vi "WebSocket FGV.vi"(0 "Tx to Server":string, 5 "Action":T2, 7 "TCP Address":string, 9 "TCP Port":u32, 11 "error in (no error)":errorcluster) -> (3 "Server Info":string, 4 "Rx from Server":string, 8 "Connection Status":bool, 13 "TxStats":T1, 14 "RxStats":T1, 15 "error out":errorcluster)   [LabVIEW 2023]
uses:
  Windows/WebSocket VIG States.ctl
  WebSocket/Stats.ctl
  WebSocket/WebSocket Stats VIG Mode.ctl
  <vilib>/Utility/error.llb/Trim Whitespace One-Sided.vi
  WebSocket/WebSocket.lvclass
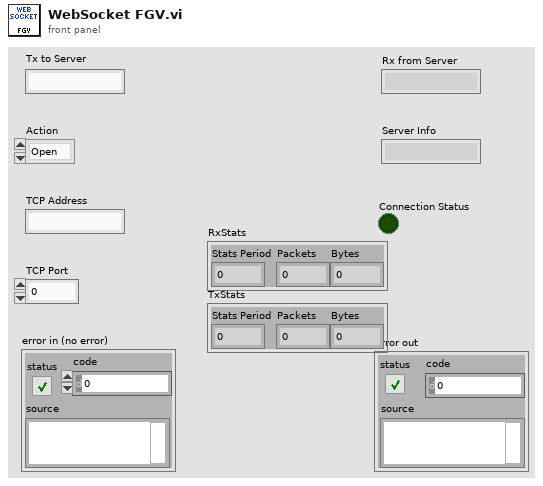
[diagram p1: front panel]
types:
  T1 = typedef "WebSocket.lvclass/Stats.ctl" = cluster{"Stats Period":dbl, "Packets":u64, "Bytes":u64}
  T2 = typedef "WebSocket VIG States.ctl" = enum16{"Open", "Close", "Send", "Receive", "Check"}
  T3 = typedef "WebSocket Stats VIG Mode.ctl" = enum16{"Init", "Set", "Update", "Get All"}
  T4 = enum16{"Standard", "Buffered", "CRLF", "Immediate"}
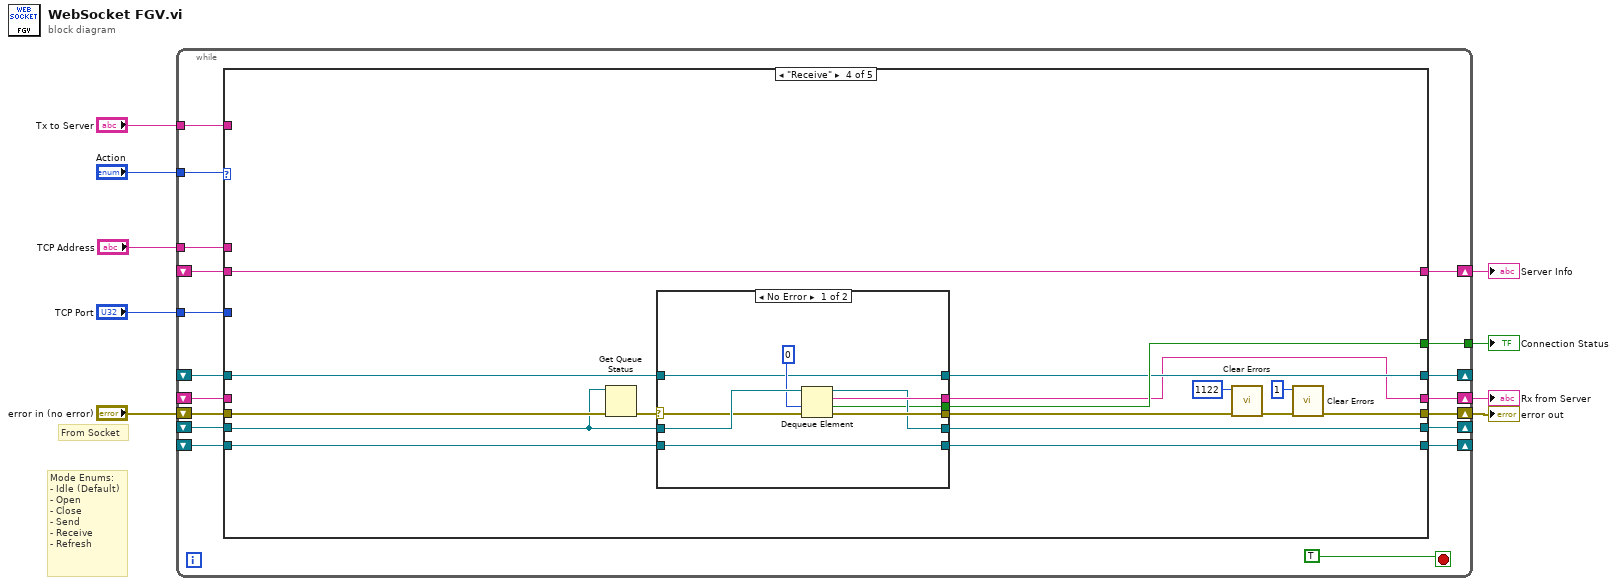
[diagram p0: block diagram]
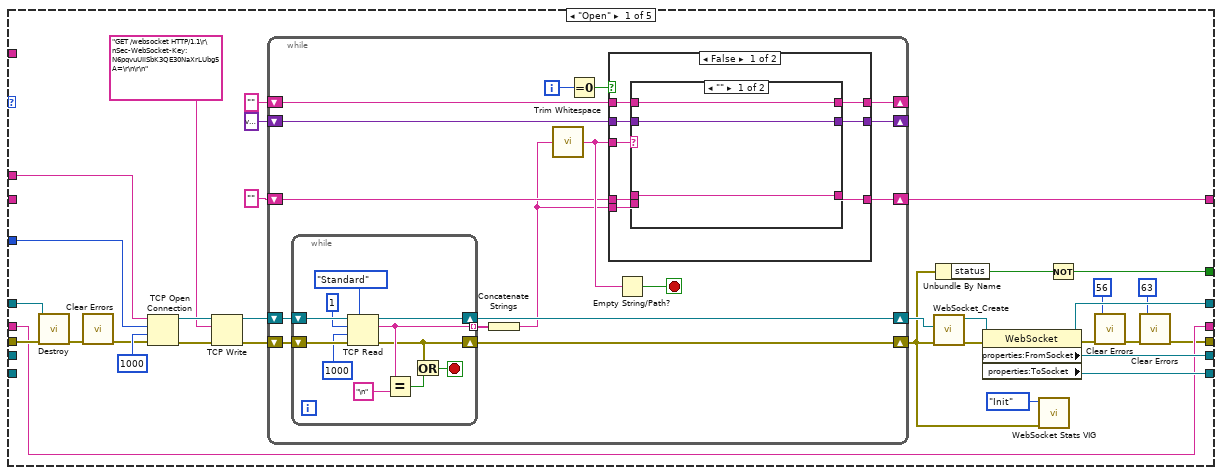
[diagram p2: hidden frame]
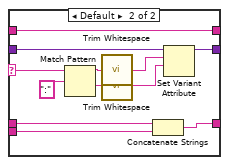
[diagram p3: hidden frame]
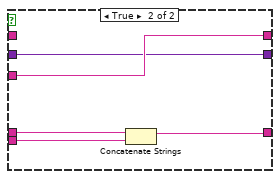
[diagram p4: hidden frame]
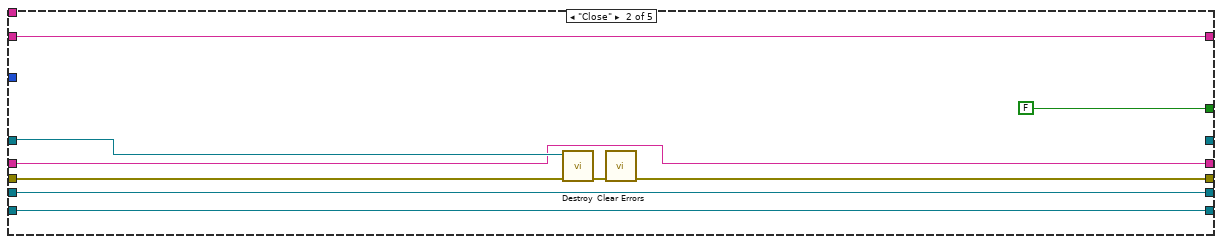
[diagram p5: hidden frame]
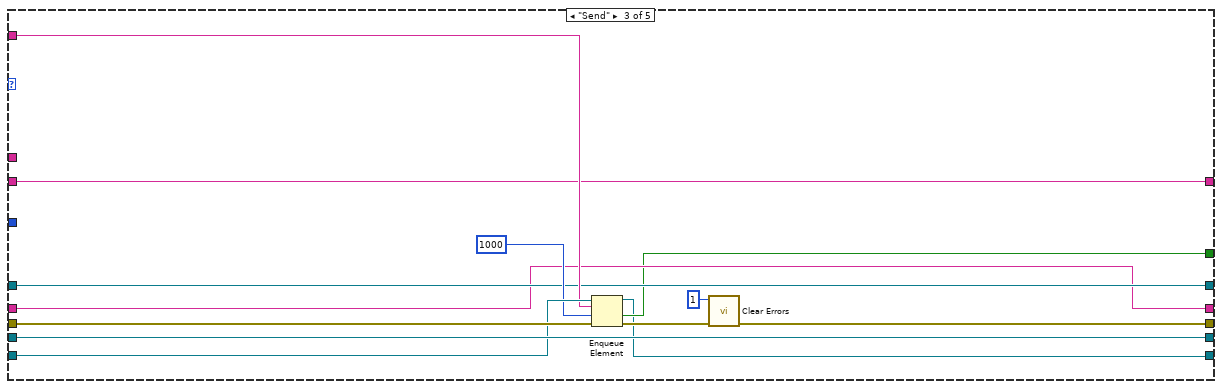
[diagram p6: hidden frame]
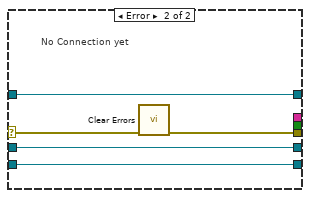
[diagram p7: hidden frame]
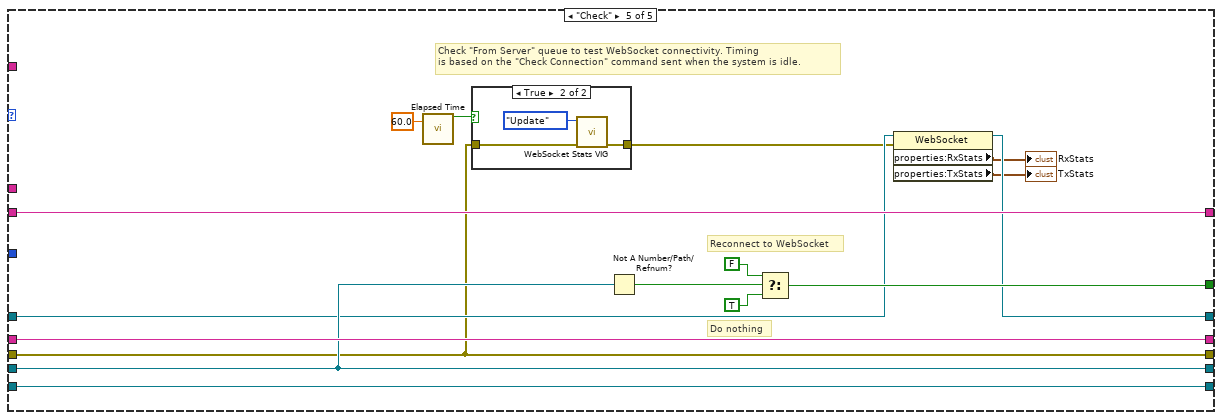
[diagram p8: hidden frame]
diagram:
  # "From Socket"
  # "Mode Enums:\n- Idle (Default)\n- Open\n- Close\n- Send\n- Receive\n- Refresh"
  n1 = while {
    tunnel: "Action" -> [w27]
    tunnel: "TCP Port" -> [w26]
    shift-right: [w24] -> w7
    shift-left: "error in (no error)" -> [w25]
    shift-right: [w23] -> _
    shift-left: _ -> [w16]
    tunnel: "TCP Address" -> [w22]
    shift-right: [w20] -> _
    shift-left: _ -> [w17]
    shift-right: [w19] -> _
    shift-left: _ -> [w18]
    tunnel: "Tx to Server" -> [w14]
    shift-right: [w21] -> w5
    shift-left: _ -> [w13]
    shift-right: [w15] -> w4
    shift-left: _ -> [w12]
    tunnel: [w10] -> w1
    stop <- TRUE stop-if-true
    n2 = case shown="\"Receive\"" w27 {
      tunnel: w26 -> [w49 _ _ _ _]
      tunnel: w25 -> [w48 w123 w135 w148 w168]
      tunnel: [w32 w115 w125 w139 w168] -> w24
      tunnel: [w34 _ w129 w144 w174] -> w23
      tunnel: w22 -> [w46 _ _ _ _]
      tunnel: [w45 w118 w130 w151 w182] -> w21
      tunnel: [w44 w119 w136 w150 w179] -> w20
      tunnel: [w43 w120 w126 w142 w180] -> w19
      tunnel: w18 -> [_ w120 w133 w143 w180]
      tunnel: w17 -> [_ w119 w136 w147 w179]
      tunnel: w16 -> [w37 w121 w129 w145 w173]
      tunnel: [w35 w117 w128 w141 w181] -> w15
      tunnel: w14 -> [_ _ w132 _ _]
      tunnel: w13 -> [_ w118 w130 w151 w182]
      tunnel: w12 -> [w35 w117 w128 _ w181]
      tunnel: [w40 FALSE ("timed out?") w127 w149 w176] -> w10
      frame "Open" {
        n3 = call-dynamic "Destroy.vi"("error in (no error)"=w48, "reference in"=w37) -> ("error out"=w38:errorcluster)  [unwired: 8 in, 1 out]
        n4 = call <vilib>:"Clear Errors.vi"("error in (no error)"=w38) -> ("error out"=w36:errorcluster)  [unwired: 5 in, 1 out]
        n5 = TCP Open Connection(address=w46, remote port or service name=w49, timeout ms (60000)=1000, error in (no error)=w36) -> (connection ID=w51:refnum<k5>, error out=w50:errorcluster)  [unwired: 1 in]
        n6 = TCP Write(connection ID=w51, data in="GET /websocket HTTP/1.1\r\nSec-WebSocket-Key: N6pqvuUIiSbK3QE30NaXrLUbg5A=\r\n\r\n", error in (no error)=w50) -> (connection ID out=w55:refnum<k5>, error out=w56:errorcluster)  [unwired: 1 in, 1 out]
        n7 = while {
          shift-right: [w67] -> _
          shift-left: variant -> [w68]
          shift-right: [w71] -> _
          shift-left: "" ("trimmed string") -> [w70]
          shift-right: [w66] -> w57
          shift-left: w55 -> [w75]
          shift-right: [w65] -> w28
          shift-left: w56 -> [w74]
          shift-right: [w63] -> w45
          shift-left: "" ("trimmed string") -> [w62]
          i -> [w73]
          stop <- w60 stop-if-true
          n8 = while {
            tunnel: [w81] -> w64 mode=indexing
            shift-right: [w82] -> w66
            shift-left: w75 -> [w86]
            shift-right: [w78] -> w65
            shift-left: w74 -> [w85]
            stop <- w77 stop-if-true
            n9 = TCP Read(connection ID=w86, bytes to read=1, error in (no error)=w85, 7:T4."Standard" ("mode (standard)"), 9:1000 ("timeout ms (25000)")) -> (connection ID out=w82:refnum<k5>, data out=w81:string, error out=w78:errorcluster)
            n10 = Equal?(x=w81, y="\n") -> (x = y?=w79:bool)
            n11 = Or(x=w78, y=w79) -> (x .or. y?=w77:bool)
          }
          n12 = Concatenate Strings(w64) -> (w61:string)
          n13 = call <vilib>:"Trim Whitespace.vi"("string"=w61) -> ("trimmed string"=w69:string)  [unwired: 1 in]
          n14 = Equal To 0?(x=w73) -> (x = 0?=w72:bool)
          n15 = case shown="False" w72 {
            tunnel: [w90 w114] -> w71
            tunnel: w69 -> [w92 w114]
            tunnel: w70 -> [w91 _]
            tunnel: w68 -> [w94 w113]
            tunnel: [w93 w113] -> w67
            tunnel: w61 -> [w89 w110]
            tunnel: [w88 w111] -> w63
            tunnel: w62 -> [w87 w112]
            frame False {
              n16 = case shown="\"\"" w92 {
                selector: w92 -> [_ w102]
                tunnel: w94 -> [w97 w106]
                tunnel: [w97 w105] -> w93
                tunnel: w91 -> [w96 w101]
                tunnel: [w96 w101] -> w90
                tunnel: w89 -> [_ w100]
                tunnel: [w95 w99] -> w88
                tunnel: w87 -> [w95 w98]
                frame "" {
                }
                frame Default {
                  n17 = Match Pattern(string=w102, regular expression=":" ("trimmed string")) -> (before substring=w107:string, after substring=w108:string)  [unwired: 1 in, 2 out]
                  n18 = call <vilib>:"Trim Whitespace.vi"("string"=w107) -> ("trimmed string"=w104:string)  [unwired: 1 in]
                  n19 = call <vilib>:"Trim Whitespace.vi"("string"=w108) -> ("trimmed string"=w103:string)  [unwired: 1 in]
                  n20 = Concatenate Strings(w98, w100) -> (w99:string)
                  n21 = Set Variant Attribute(Variant=w106, name=w104, value=w103) -> (Variant out=w105:variant)  [unwired: 1 in, 2 out]
                }
              }
            }
            frame True {
              n22 = Concatenate Strings(w112, w110) -> (w111:string)
            }
          }
          n23 = Empty String/Path?(string/path=w69) -> (empty?=w60:bool)
        }
        n24 = call "WebSocket_Create.vi"("error in (no error)"=w28, "Socket"=w57) -> ("error out"=w59:errorcluster, "reference out"=w58:refnum<class "WebSocket.lvclass">)  [unwired: 8 in]
        n25 = Unbundle By Name(w28) -> ("status"=w41:bool)
        n26 = property class="WebSocket"(reference=w58, error in=w59) -> (reference out=w34:refnum<class "WebSocket.lvclass">, error out=w47:errorcluster, "properties:FromSocket"=w44:refnum<queue>, "properties:ToSocket"=w43:refnum<queue>)
        n27 = call "WebSocket Stats VIG.vi"("error in (no error)"=w28, "mode"=WebSocket_Stats_VIG_Mode."Init") -> ()  [unwired: 7 in, 3 out]
        n28 = Not(x=w41) -> (.not. x?=w40:bool)
        n29 = call <vilib>:"Clear Errors.vi"("error in (no error)"=w47, "specific error code to clear (0: all)"=56) -> ("error out"=w33:errorcluster)  [unwired: 4 in, 1 out]
        n30 = call <vilib>:"Clear Errors.vi"("error in (no error)"=w33, "specific error code to clear (0: all)"=63) -> ("error out"=w32:errorcluster)  [unwired: 4 in, 1 out]
      }
      frame "Close" {
        n31 = call-dynamic "Destroy.vi"("error in (no error)"=w123, "reference in"=w121) -> ("error out"=w122:errorcluster)  [unwired: 8 in, 1 out]
        n32 = call <vilib>:"Clear Errors.vi"("error in (no error)"=w122) -> ("error out"=w115:errorcluster)  [unwired: 5 in, 1 out]
      }
      frame "Send" {
        n33 = Enqueue Element(queue=w133, element=w132, timeout in ms (-1)=1000, error in (no error)=w135) -> (queue out=w126:refnum<queue>, timed out?=w127:bool, error out=w134:errorcluster)
        n34 = call <vilib>:"Clear Errors.vi"("error in (no error)"=w134, "specific error code to clear (0: all)"=1) -> ("error out"=w125:errorcluster)  [unwired: 4 in, 1 out]
      }
      frame "Receive" {
        n35 = Get Queue Status(queue=w147, error in (no error)=w148) -> (error out=w146:errorcluster)  [unwired: 1 in, 7 out]
        n36 = case shown="No Error" w146 {
          selector: w146 -> [w155 w163]
          tunnel: [w161 w162] -> w152
          tunnel: w147 -> [w160 w166]
          tunnel: [w159 _] -> w141
          tunnel: [w157 w166] -> w150
          tunnel: [w156 _] -> w149
          tunnel: w145 -> [w154 w164]
          tunnel: [w154 w164] -> w144
          tunnel: w143 -> [w153 w165]
          tunnel: [w153 w165] -> w142
          frame No Error {
            n37 = Dequeue Element(queue=w160, timeout in ms (-1)=0, error in (no error)=w155) -> (queue out=w157:refnum<queue>, element=w159:string, timed out?=w156:bool, error out=w161:errorcluster)
          }
          frame Error {
            # "No Connection yet"
            n38 = call <vilib>:"Clear Errors.vi"("error in (no error)"=w163) -> ("error out"=w162:errorcluster)  [unwired: 5 in, 1 out]
          }
        }
        n39 = call <vilib>:"Clear Errors.vi"("error in (no error)"=w152, "specific error code to clear (0: all)"=1122) -> ("error out"=w140:errorcluster)  [unwired: 4 in, 1 out]
        n40 = call <vilib>:"Clear Errors.vi"("error in (no error)"=w140, "specific error code to clear (0: all)"=1) -> ("error out"=w139:errorcluster)  [unwired: 4 in, 1 out]
      }
      frame "Check" {
        # "Check \"From Server\" queue to test WebSocket connectivity. Timing\nis based on the \"Check Connection\" command sent when the system is idle."
        # "Reconnect to WebSocket"
        # "Do nothing"
        n41 = call "Elapsed Time.vi"("Elapsed Time Target"=60.0) -> ("Time has Elapsed"=w169:bool)  [unwired: 13 in, 5 out]
        n42 = case shown="True" w169 {
          tunnel: w168 -> [w183 w185]
          tunnel: [w183 w184] -> w167
          frame False {
          }
          frame True {
            n43 = call "WebSocket Stats VIG.vi"("error in (no error)"=w185, "mode"=WebSocket_Stats_VIG_Mode."Update") -> ("error out"=w184:errorcluster)  [unwired: 7 in, 2 out]
          }
        }
        n44 = Not A Number/Path/Refnum?(number/path/refnum=w179) -> (NaN/Path/Refnum?=w178:bool)
        n45 = Select(t=FALSE, s=w178, f=TRUE) -> (s? t:f=w176:bool)
        n46 = property class="WebSocket"(reference=w173, error in=w167) -> (reference out=w174:refnum<class "WebSocket.lvclass">, "properties:RxStats"=→"RxStats":T1, "properties:TxStats"=→"TxStats":T1)  [unwired: 1 out]
      }
    }
  }
  "error out" <- w7
  "Server Info" <- w5
  "Rx from Server" <- w4
  "Connection Status" <- w1
